vi "Update Card Simulator Control.vi"(8 "error in (no error)":errorcluster, 10 "ATM State":T1, 11 "ATM View Model in":refnum<class "ATM View Model.lvclass">) -> (0 "error out":errorcluster)   [LabVIEW 2020, in "ATM View Model.lvclass"]
uses:
  ATM View Model.lvclass
  ATM Controller/State.ctl
  Controls.ctl
  ATM View Model.lvclass/ATM View Model.ctl
  ATM Controller/ATM Controller.lvclass
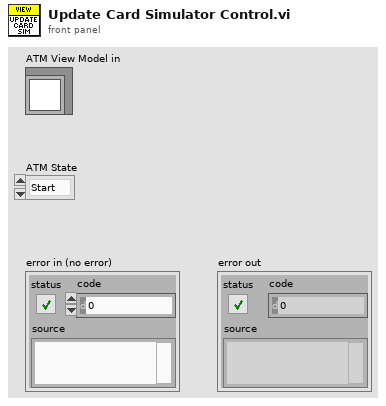
[diagram p1: front panel]
types:
  T1 = typedef "ATM Controller.lvclass/State.ctl" = enum16{"Start", "Card Inserted", "Verification Failed", "Verification Succeeded", "Depositing", "Depositing Completed", "Withdrawing", "Withdraw Completed", "Withdraw Failed", "Balance Inquiry", "Terminate"}
  T2 = typedef "ATM View Model.lvclass/Controls.ctl" = enum16{"User Input", "Enter", "Left Menu", "Right Menu", "Left Button", "Right Button", "Card Simulator"}
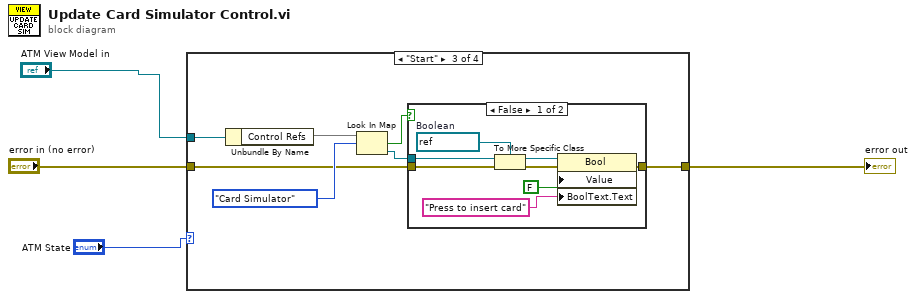
[diagram p0: block diagram]
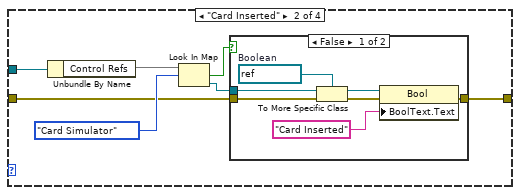
[diagram p3: hidden frame]
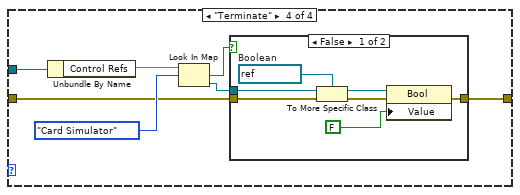
[diagram p6: hidden frame]
diagram:
  n1 = case shown="\"Start\"" "ATM State" {
    tunnel: [w5 w11 w26 w42] -> w4
    tunnel: "ATM View Model in" -> [_ w7 w22 w38]
    tunnel: "error in (no error)" -> [w5 w6 w21 w37]
    frame Default {
    }
    frame "Card Inserted" {
      n2 = Unbundle By Name(w7) -> ("Control Refs"=w8:map{T2, refnum<vi>})
      n3 = Look In Map(map=w8, key=Controls."Card Simulator") -> (key not found?=w12:bool, value=w10:refnum<vi>)  [unwired: 1 in]
      n4 = case shown="False" w12 {
        tunnel: w6 -> [w19 w20]
        tunnel: w10 -> [w17 _]
        tunnel: [w15 w20] -> w11
        frame False {
          w16 = refnum<vi> refnum  # Boolean
          n5 = To More Specific Class(target class=w16, reference=w17, error in=w19) -> (specific class reference=w14:refnum<vi>, error out=w18:errorcluster)
          n6 = property class="Bool"(reference=w14, error in=w18, "BoolText.Text"="Card Inserted" ("Boolean Text.Text")) -> (error out=w15:errorcluster)  [unwired: 1 out]
        }
        frame True {
        }
      }
    }
    frame "Start" {
      n7 = Unbundle By Name(w22) -> ("Control Refs"=w23:map{T2, refnum<vi>})
      n8 = Look In Map(map=w23, key=Controls."Card Simulator") -> (key not found?=w27:bool, value=w25:refnum<vi>)  [unwired: 1 in]
      n9 = case shown="False" w27 {
        tunnel: w21 -> [w35 w36]
        tunnel: w25 -> [w33 _]
        tunnel: [w31 w36] -> w26
        frame False {
          w32 = refnum<vi> refnum  # Boolean
          n10 = To More Specific Class(target class=w32, reference=w33, error in=w35) -> (specific class reference=w30:refnum<vi>, error out=w34:errorcluster)
          n11 = property class="Bool"(reference=w30, error in=w34, "Value"=FALSE, "BoolText.Text"="Press to insert card" ("Boolean Text.Text")) -> (error out=w31:errorcluster)  [unwired: 1 out]
        }
        frame True {
        }
      }
    }
    frame "Terminate" {
      n12 = Unbundle By Name(w38) -> ("Control Refs"=w39:map{T2, refnum<vi>})
      n13 = Look In Map(map=w39, key=Controls."Card Simulator") -> (key not found?=w43:bool, value=w41:refnum<vi>)  [unwired: 1 in]
      n14 = case shown="False" w43 {
        tunnel: w37 -> [w50 w51]
        tunnel: w41 -> [w48 _]
        tunnel: [w46 w51] -> w42
        frame False {
          w47 = refnum<vi> refnum  # Boolean
          n15 = To More Specific Class(target class=w47, reference=w48, error in=w50) -> (specific class reference=w45:refnum<vi>, error out=w49:errorcluster)
          n16 = property class="Bool"(reference=w45, error in=w49, "Value"=FALSE) -> (error out=w46:errorcluster)  [unwired: 1 out]
        }
        frame True {
        }
      }
    }
  }
  "error out" <- w4
